vi "test_LocationFGV_GetLocation_LocationResolved.vi"(8 "error in":errorcluster) -> (0 "error out":errorcluster, 2 "result":string, 3 "pass":bool)   [LabVIEW 2020, in "MeasurementServerTests.lvlib" / "Discovery Tests.lvlib"]
uses:
  Discovery Tests.lvlib
  Fake Service Location Generator Action.ctl
  Runtime/APIs/Discovery V1/TypeDefs/Service Location FGV Action.ctl
  Runtime/APIs/Discovery V1/Plug-In SDK Discovery V1 API.lvlib
  gRPC/Generated APIs/ni/measurementlink/discovery/v1/RPC Messages/ni_measurementlink_discovery_v1_ResolveServiceRequest.ctl
  gRPC/Generated APIs/ni/measurementlink/discovery/v1/ni.measurementlink.discovery.v1.lvlib
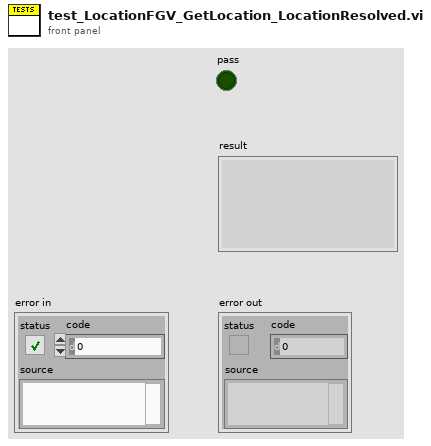
[diagram p1: front panel]
types:
  T1 = typedef "ni.measurementlink.discovery.v1.lvlib/ni_measurementlink_discovery_v1_ResolveServiceRequest.ctl" = cluster{"provided_interface":string, "service_class":string}
  T2 = typedef "Plug-In SDK Discovery V1 API.lvlib/Service Location FGV Action.ctl" = enum16{"Get Service Location", "Reresolve Service Location"}
  T3 = typedef "MeasurementServerTests.lvlib/Discovery Tests.lvlib/Fake Service Location Generator Action.ctl" = enum16{"Generate New Location", "Reset", "Error on Next Call"}
  T4 = typedef "ni.measurementlink.discovery.v1.lvlib/ni_measurementlink_discovery_v1_ServiceLocation.ctl" = cluster{"location":string, "insecure_port":string, "ssl_authenticated_port":string}
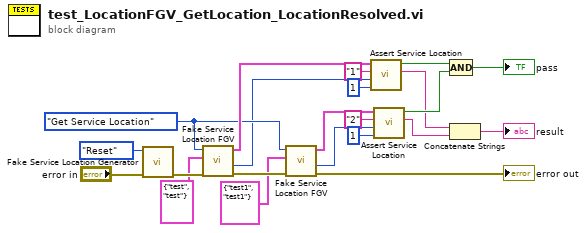
[diagram p0: block diagram]
diagram:
  w14 = Service_Location_FGV_Action."Get Service Location" ("action")
  n1 = call "Fake Service Location Generator.vi"("error in"="error in", "action"=Fake_Service_Location_Generator_Action."Reset") -> ("error out"=w21:errorcluster)  [unwired: 8 in, 1 out]
  n2 = call "Fake Service Location FGV.vi"("error in"=w21, "resolve service request"=T1 {"provided_interface"="test", "service_class"="test"}, "action"=w14) -> ("error out"=w17:errorcluster, "unique id out"=w12:u64, "service location"=w19:T4)  [unwired: 6 in]
  n3 = call "Fake Service Location FGV.vi"("error in"=w17, "resolve service request"=T1 {"provided_interface"="test1", "service_class"="test1"}, "action"=w14) -> ("error out"=→"error out":errorcluster, "unique id out"=w8:u64, "service location"=w10:T4)  [unwired: 6 in]
  n4 = call "Assert Service Location.vi"("expected unique id"=u64 1, "actual unique id"=w12, "expected service location port"="1", "actual service location"=w19) -> ("result"=w3:string, "pass"=w5:bool)  [unwired: 6 in]
  n5 = call "Assert Service Location.vi"("expected unique id"=u64 1, "actual unique id"=w8, "expected service location port"="2", "actual service location"=w10) -> ("result"=w1:string, "pass"=w6:bool)  [unwired: 6 in]
  n6 = Compound Arithmetic op=AND(w5, w6) -> (→"pass":bool)
  n7 = Concatenate Strings(w3, w1) -> (→"result":string)
